vi "Run Test - Save Report (SubVI).vi"(8 "error in (no error)":errorcluster, 11 "Cluster":T1 {"M Event" items=["Stop", "Running", "PID", "Up Limit", "Down Limit", "Load Limit"]; "Test Type" items=["Please Select", "Triaxial Shear", "Triaxial UU", "Shearbox", "Permeability", "Consolidation (Stepped Loading)/Swelling", "Saturation (Incremental)", "User Defined", "UCT", "Isotropic Consolidation", "Swelling Pressure"]; "Data"."Test Type" items=["Please Select", "Triaxial Shear", "Triaxial UU", "Shearbox", "Permeability", "Consolidation (Stepped Loading)/Swelling", "Saturation (Incremental)", "User Defined", "UCT", "Isotropic Consolidation", "Swelling Pressure"]}) -> (0 "error out":errorcluster)   [LabVIEW 2019]
uses:
  Controls/RunTest - Data Structure.ctl
  Controls/Test Panel - Data Structure.ctl
  Controls/Station - Test Type.ctl
  <vilib>/Utility/miscctls.llb/LVRowAndColumnTypeDef.ctl
  Controls/RunTest - Calculate Data.ctl
  <vilib>/httpClient/ClientHandle.ctl
  Controls/RunTest - Start Condition.ctl
  Controls/RunTest - Stop Condition.ctl
  Controls/UDP - Event.ctl
  <vilib>/httpClient/LabVIEWHTTPClient.lvlib
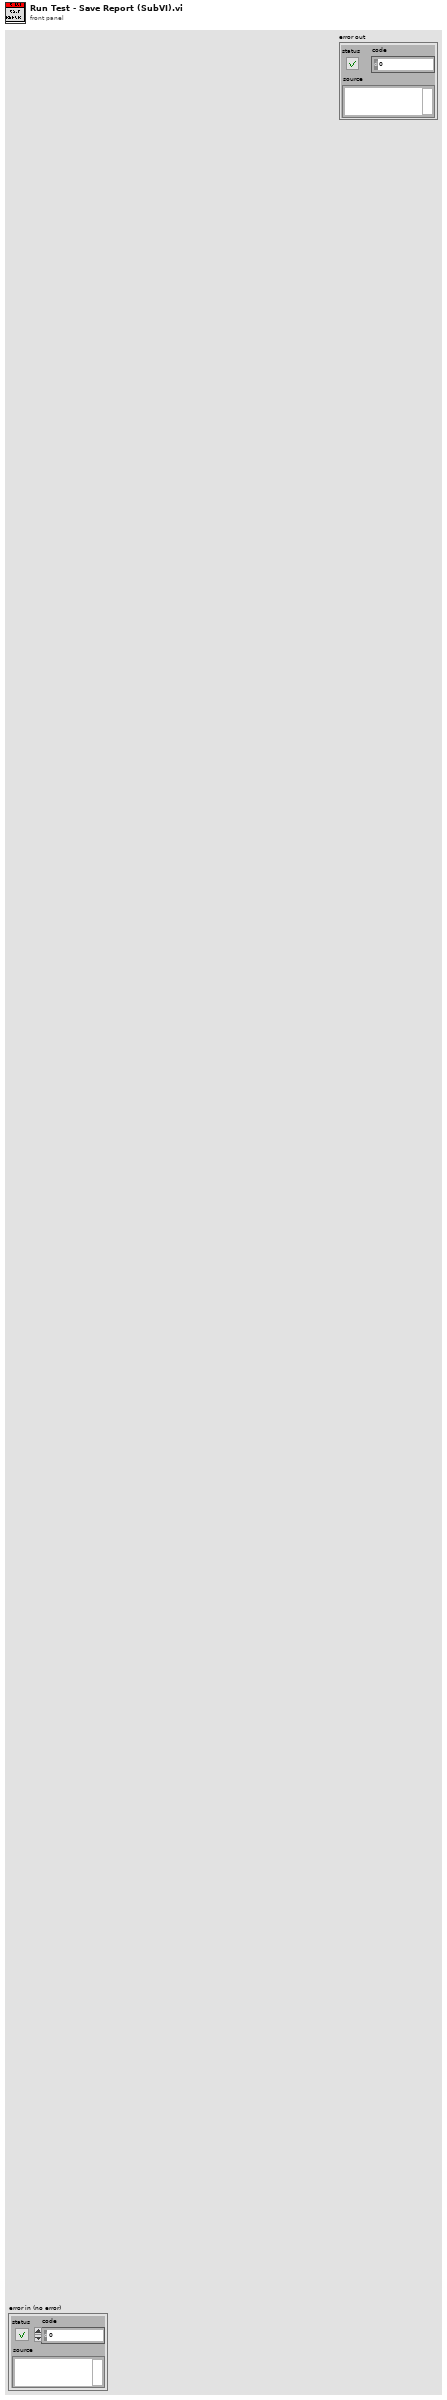
[diagram p1: front panel]
types:
  T1 = typedef "RunTest - Data Structure.ctl" = cluster{"Test Plan":string[], "PlanRow":i32, "Device Name":string[], "Timeout":i32, "Start?":bool, "Pause?":bool, "IP Address":string[], "LogRow":i32, "Logtype":u16, "Log Elapse":sgl, "Data":T2, "Stop log?":bool, "tdms":refnum<k34>, "Sensor Data":sgl[], "Start time":timestamp, "Prev Log Elapse":u32, "Plot":u16, "X-Axis":u16[], "Y-Axis":u16[], "XY":cluster{"X":dbl, "Y":dbl}[][], "End Stage?":bool, "1run":bool, "Condition":u16[], "Start Con":bool, "Log Con":bool, "Stop Con":bool, "Start Elapse":dbl, "Start Load":dbl, "Motor":i32, "StartRow":i32, "number log":i32, "Dir":bool, "Start time test":timestamp, "Auto":bool, "Check return?":bool, "Inv":cluster{"M":i32[], "Bool":bool[]}, "tdms temp":refnum<k34>, "Zero?":bool, "Plot Timer":dbl, "1st Run":bool, "TDMS Path":path, "MaxLoad":dbl, "Log Timer":sgl[], "Test Type":T3, "Log Sensor":string[], "Save?":bool, "1st Log":bool, "Y-Axis 2":u16[], "On Y-Axis 2":bool, "Decimal":u8[], "Init":cluster{"PWP TS":sgl, "Load TS":sgl, "Volume TS":sgl, "Disp TS":sgl, "CP":sgl, "Vol In":sgl, "Vol Out":sgl, "Load UCT":sgl, "Disp UCT":sgl, "PWP Sat":sgl, "CP Sat":sgl, "Volume IsoCons":sgl, "PWP IsoCons":sgl, "PWP TUU":sgl, "Load TUU":sgl, "Volume TUU":sgl, "Disp TUU":sgl, "Load Cons":sgl, "Disp Cons":sgl, "Volume Sat":sgl, "Vertical Load SB":sgl, "Vertical Disp SB":sgl, "H Disp SB":sgl, "H Load SB":sgl}, "Calc":T5, "Device Index":i32[], "Channel Index":i32[], "http ref":T6, "fileid":string, "Step Cons":cluster{"V Stress":sgl, "H Settlement":sgl}, "RunTest":bool, "Graph Last":i32, "Init?":bool, "Datalog":bool[], "Start":T7, "Stop":T8, "Running?":bool, "StartTime":dbl, "Log Prev Time":dbl, "KeyName":string[], "Test RunTime":dbl, "Log Prev Axial":dbl, "M Event":T9[], "Last Log":bool, "popup":bool, "PreStart UU":bool, "PreStart Sat":bool}
  T2 = typedef "Test Panel - Data Structure.ctl" = cluster{"Station":string, "Sample ID":string, "Job No":string, "Job Description":string, "Filename":string, "Test Type":T3, "Speciment No":string, "Depth":string, "Height":string, "Diameter/Length":string, "Weight":string, "Test Parameter":string, "Station[]":string[], "Edit Pos":T4, "Edit Pos Prev":T4, "Area":string, "Path":string}
  T3 = typedef "Station - Test Type.ctl" = u16
  T4 = typedef "LVRowAndColumnTypeDef.ctl" = cluster{"Row":i32, "Column":i32}
  T5 = typedef "RunTest - Calculate Data.ctl" = cluster{"TS":cluster{"Change PWP":sgl, "Change Vol":sgl, "Axial Load":sgl, "CiL":sgl, "Deviator":sgl, "Axial Strain":sgl, "MaxDeviator":sgl}, "TUU":cluster{"Change PWP":sgl, "Axial Load":sgl, "CiL":sgl, "Deviator":sgl, "Axial Strain":sgl, "MaxDeviator":sgl}, "Sat":cluster{"B Value":sgl, "PWP Diss":sgl, "CPP":sgl, "CV":sgl}, "Per":cluster{"Change Vol In":sgl, "Change Vol Out":sgl, "Mean Vol":sgl, "Gradient Pressure":sgl, "Outlet Flow":sgl, "Inlet Flow":sgl, "I X1":sgl, "I X2":sgl, "I Y1":sgl, "I Y2":sgl, "O X1":sgl, "O X2":sgl, "O Y1":sgl, "O Y2":sgl}, "Step Cons":cluster{"V Stress":sgl, "H Settlement":sgl, "Total H Settle":sgl, "Prev Total H":sgl}, "UCT":cluster{"ALC":sgl, "H Change":sgl, "Deviator":sgl, "Axial Strain":sgl, "V Stress":sgl, "MaxDeviator":sgl}, "ISO Cons":cluster{"CPP":sgl, "PWP Diss":sgl, "CV":sgl}, "SB":cluster{"Speci LenC":sgl, "Shear Strain":sgl, "H LC":sgl, "Normal Stress":sgl, "Shear Stress":sgl, "MaxShear":sgl}}
  T6 = typedef "LabVIEWHTTPClient.lvlib/ClientHandle.ctl" = refnum<k1>
  T7 = typedef "RunTest - Start Condition.ctl" = cluster{"Cons":cluster{"VS":dbl, "Delay":bool, "No Delay":dbl}, "Sat":cluster{"CP":dbl, "BP":dbl, "StartBP":bool, "Target CP":bool, "Target BP":bool}, "Iso":cluster{"BP":dbl}, "TS":cluster{"SS":dbl, "Engage":bool, "ES":dbl, "LC":dbl, "PreStart":bool, "Trig SS":bool, "Drain":dbl}, "TUU":cluster{"SS":dbl, "Engage":bool, "ES":dbl, "LC":dbl, "PreStart":bool, "Trig SS":bool, "CP":dbl, "Delay Value":dbl, "Delay":bool, "CP PID":bool}, "UCT":cluster{"SS":dbl, "Engage":bool, "ES":dbl, "LC":dbl, "PreStart":bool, "Trig SS":bool}, "Enable?":bool, "SB":cluster{"SS":dbl, "Engage":bool, "ES":dbl, "LC":dbl, "PreStart":bool, "Trig SS":bool, "VS":dbl, "Delay Value":dbl, "Delay":bool, "VS PID":bool}, "Perm":cluster{"DP":dbl}}
  T8 = typedef "RunTest - Stop Condition.ctl" = cluster{"Cons":cluster{"Select":i32, "Disp":dbl, "Time":dbl, "Time2":dbl, "Disp 2":dbl, "Time Cond":dbl, "Last Disp":dbl, "Swell":bool}, "Sat":cluster{"Select":i32, "PP":dbl, "Time":dbl, "VC":dbl, "Time2":dbl, "Time Cond":dbl, "Last PP":dbl, ".B":bool, "B":dbl, "Last Vc":dbl, "Time Cond 2":dbl, "Time3":dbl, "Time Cond 3":dbl}, "Iso":cluster{"PP":dbl, "Time":dbl, "VC":dbl, "Time2":dbl, "Time Cond":dbl, "Last Vc":dbl, ".PP":bool, "Time Cond 2":dbl, "Select":i32}, "TS":cluster{"Axial":dbl, ".MaxDev":bool, "MaxDev Value":dbl, "Return":bool, "Reset":bool, "Prev Time":dbl, "PostStop Run":bool, "CP Stop":bool, "BP Stop":bool, "PostStop Trig":bool, "Reset Value":dbl, "BPTrig":bool, "CPTrig":bool, "VLCTrig":bool}, "TUU":cluster{"Axial":dbl, ".MaxDev":bool, "MaxDev Value":dbl, "Return":bool, "Reset":bool, "Prev Time":dbl, "PostStop Run":bool, "CP Stop":bool, "BP Stop":bool, "PostStop Trig":bool, "Reset Value":dbl, "BPTrig":bool, "CPTrig":bool, "VLCTrig":bool}, "UCT":cluster{"Axial":dbl, ".MaxDev":bool, "MaxDev Value":dbl, "Return":bool, "Reset":bool, "Prev Time":dbl, "PostStop Run":bool, "CP Stop":bool, "BP Stop":bool, "PostStop Trig":bool}, "Enable?":bool, "SB":cluster{"Shear":dbl, ".MaxShear":bool, "MaxShear Value":dbl, "Return":bool, "Reset":bool, "Prev Time":dbl, "PostStop Run":bool, "CP Stop":bool, "BP Stop":bool, "PostStop Trig":bool, "Reset Value":dbl, "BPTrig":bool, "CPTrig":bool, "VLCTrig":bool}, "Perm":cluster{"Max Time":bool, "Reset":bool, "PostStop Run":bool, "Ratio":bool, "Reset Value":dbl, "Time":dbl, "RatioTime":dbl, "RatioMore":dbl, "RatioLess":dbl, "Time Cond":dbl, "Time Cond 2":dbl, "Prev IF":dbl, "Prev OF":dbl, "PostStop Trig":bool, "BP Trig":bool, "DP Stop":bool, "BP Stop":bool, "CP Stop":bool, "CP Trig":bool}, "SP":cluster{".Max Time":bool, ".Time":bool, "Time":dbl, "MaxTime":dbl, "Time Cond":dbl, "Max Time Cond":dbl, "Stress":dbl}}
  T9 = typedef "UDP - Event.ctl" = u16
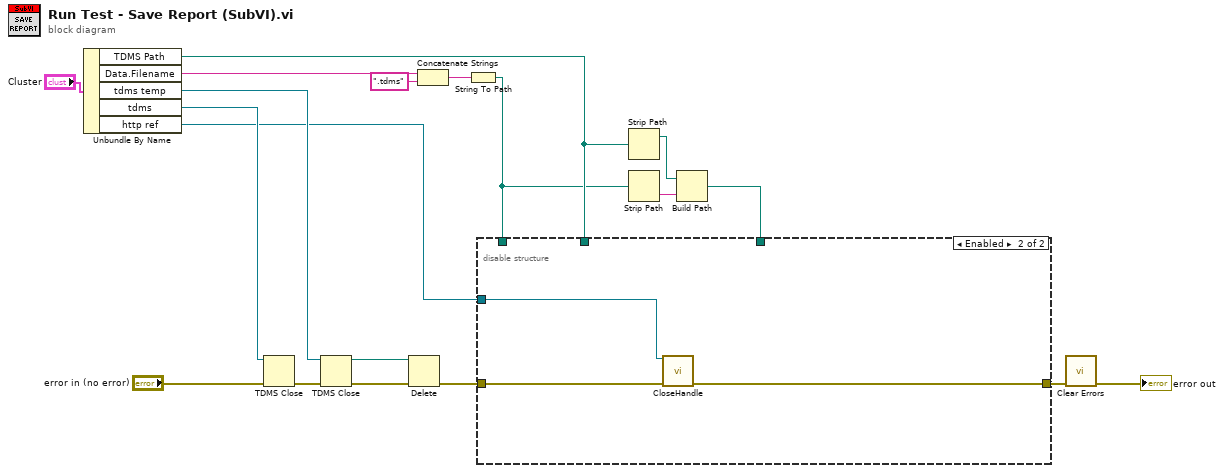
[diagram p0: block diagram]
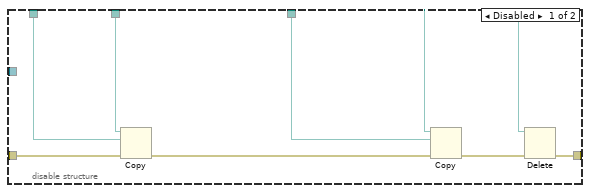
[diagram p2: hidden frame]
diagram:
  n1 = Unbundle By Name("Cluster") -> ("TDMS Path"=w14:path, "Data.Filename"=w1:string, "tdms temp"=w16:refnum<k34>, "tdms"=w15:refnum<k34>, "http ref"=w2:T6)
  n2 = TDMS Close(8:"error in (no error)", 11:w15) -> (0:w13:errorcluster)  [unwired: 1 out]
  n3 = TDMS Close(8:w13, 11:w16) -> (0:w6:errorcluster, 3:w4:path)
  n4 = Delete(path (use dialog)=w4, error in=w6) -> (error out=w5:errorcluster)  [unwired: 3 in, 2 out]
  n5 = Concatenate Strings(w1, ".tdms" ("string")) -> (w11:string)
  n6 = String To Path(string=w11) -> (path=w10:path)
  n7 = Strip Path(path=w14) -> (stripped path=w9:path)  [unwired: 1 out]
  n8 = Strip Path(path=w10) -> (name=w8:string)  [unwired: 1 out]
  n9 = Build Path(base path=w9, name or relative path=w8) -> (appended path=w7:path)
  n10 = disable-structure shown="Enabled" {
    disable-tunnel: [w26 w28] -> w17
    disable-tunnel: w14 -> [w25 _]
    disable-tunnel: w10 -> [w23 _]
    disable-tunnel: w7 -> [w22 _]
    disable-tunnel: w5 -> [w20 w29]
    disable-tunnel: w2 -> [_ w27]
    frame Disabled {
      n11 = Copy(8:w20, 10:w23, 11:w25) -> (0:w24:errorcluster)  [unwired: 2 in, 2 out]
      n12 = Copy(8:w24, 10:w22, 11:w25) -> (0:w21:errorcluster)  [unwired: 2 in, 2 out]
      n13 = Delete(path (use dialog)=w25, error in=w21) -> (error out=w26:errorcluster)  [unwired: 3 in, 2 out]
    }
    frame Enabled {
      n14 = call <vilib>:"CloseHandle.vi"("client handle"=w27, "error in (no error)"=w29) -> ("error out"=w28:errorcluster)  [unwired: 13 in]
    }
  }
  n15 = call <vilib>:"Clear Errors.vi"("error in (no error)"=w17) -> ("error out"=→"error out":errorcluster)  [unwired: 5 in, 1 out]
